vi "FFT.vi"() -> ()   [LabVIEW 2020]
uses:
  <vilib>/rvi/Analysis/measure/FFT/simModelSupport/niFPGA FFT Outside SCTL Sim Properties.ctl
  <vilib>/rvi/Analysis/measure/FFT/simModelSupport/niFPGA FFT Sim Types.ctl
  <vilib>/rvi/Analysis/measure/FFT/simModelSupport/niFpgaFFTSimArithmeticProperties.ctl
  <vilib>/rvi/Analysis/measure/FFT/simModelSupport/niFpgaFFTSimDfxp.ctl
  <vilib>/fxp/LVFixedPointQuantizationPolicyTypeDef.ctl
  <vilib>/rvi/FXPMathLib/FxpAtan2/subVIs/nifxpmath_Atan2_SimConfig.ctl
  <vilib>/rvi/FXPMathLib/FxpSinAndCos/subVIs/nifxpmath_SinAndCos_SimConfig.ctl
  <vilib>/rvi/DataTransferAndStorage/Container/Common/niFpgaContainerGetUniqueNameForEmu.vi
  <vilib>/rvi/DataTransferAndStorage/Container/Common/niFpgaContainerSetEmuInfo.vi
  <vilib>/rvi/eio/common/nirviEmuReportErrorAndStop.vi
  <vilib>/rvi/interface/RandomDataEmulation/niFpgaRandomDataHandleErrors.vi
  <vilib>/rvi/DataTransferAndStorage/Container/Common/niFpgaContainerExecOnDevCompGetState.vi
  <vilib>/rvi/Emulation/niFpgaEmulationIsFPGAContextNoSignature.vi
  <vilib>/rvi/Emulation/niFpgaSctlEmulationGetInTimedLoop.vi
  <vilib>/rvi/errors/niFpgaSetErrorForExecOnDevCompSimple.vi
  <vilib>/rvi/FIFO/Fifo_Resource/nirvififoEmulationSetSize.vi
  <vilib>/rvi/FIFO/Fifo_Resource/nirviFifoEmulationQueueMgr.vi
  <instcachedir>/0/nirviFifoEmulationQueueMgr_E5CAEC123FF24DC58D834DCA3CDAA9B5.lvgen/nirviFifoEmulationQueueMgr_E5CAEC123FF24DC58D834DCA3CDAA9B5_008.vi
  <vilib>/rvi/FIFO/Fifo_Resource/nirvififoEmulationDetermineInputValidOut.vi
  <vilib>/rvi/FIFO/Fifo_Resource/nirvififoEmulationCreateLock.vi
  <vilib>/rvi/Emulation/niFpgaProcessEmulError.vi
  <vilib>/rvi/FIFO/Fifo_Resource/nirvififoEmulationObtainLock.vi
  <vilib>/rvi/FIFO/Fifo_Resource/nirvififoEmulationReleaseLock.vi
  <vilib>/rvi/occurrence/nirviWaitOnOccurrenceBase.vi
  <vilib>/rvi/errors/nirviReportUnexpectedCaseInternalError.vi
  <vilib>/rvi/errors/nirviReportUnexpectedCaseInternalError (U32).vi
  <vilib>/Utility/error.llb/Clear Errors.vi
  <vilib>/rvi/Emulation/niFpgaGetClockAttributes.vi
  <vilib>/rvi/Emulation/niFpgaEmulationReportErrorSimple.vi
  <vilib>/rvi/Analysis/measure/FFT/simModelSupport/niFpgaFFTSimModelOutsideSCTLCore.vi
  <vilib>/rvi/FXPMathLib/FxpAtan2/simVIs/DllFxpAtan2Temp_sub.vi
  <instcachedir>/0/nirviFifoEmulationQueueMgr_E5CAEC123FF24DC58D834DCA3CDAA9B5.lvgen/nirviFifoEmulationQueueMgr_E5CAEC123FF24DC58D834DCA3CDAA9B5_002.vi
  <instcachedir>/0/nirviFifoEmulationQueueMgr_E5CAEC123FF24DC58D834DCA3CDAA9B5.lvgen/nirviFifoEmulationQueueMgr_E5CAEC123FF24DC58D834DCA3CDAA9B5_004.vi
  <vilib>/rvi/Emulation/niFpgaCriticalErrorInLSC.vi
  <vilib>/rvi/FXPMathLib/FxpSinAndCos/simVIs/DllFxpSinAndCosTemp_sub.vi
  <vilib>/rvi/LocalResourceManager/LocalResourceManager.xnode
  <vilib>/rvi/DataTransferAndStorage/Container/XNode/niFpgaContainer.xnode
  <vilib>/rvi/interface/RandomDataEmulation/nirviRandomDataFpgaReadWriteTemplate.vi
  <vilib>/rvi/FIFO/Fifo_Resource/niFpgaFifoEmulationRefIn.vi
  <vilib>/rvi/Analysis/measure/FFT/XNode/niFpgaFFT.xnode
  <vilib>/rvi/FXPMathLib/FxpAtan2/XNode/nifxpmath_Atan2.xnode
  <vilib>/rvi/FXPMathLib/FxpSinAndCos/XNode/nifxpmath_SinAndCos.xnode
panel:
  out "Array":fxp<+/-,33,17>[](array[numeric])
  out "x*y":fxp<+/-,32,16>[](array[numeric])
  out "Numeric 4":i32
  out "Numeric 2":i32
  out "Numeric 3":i32
  out "val":fxp<+,64,48>
  out "n*d":fxp<+,32,16>
  out "size(s)":i32
  out "N":fxp<+/-,18,17>
  in  "n":fxp<+,32,16>
  in  "s (sample rate)":fxp<+,32,16>
  out "Numeric":i32
  # "n=512"
  # "s=51200"
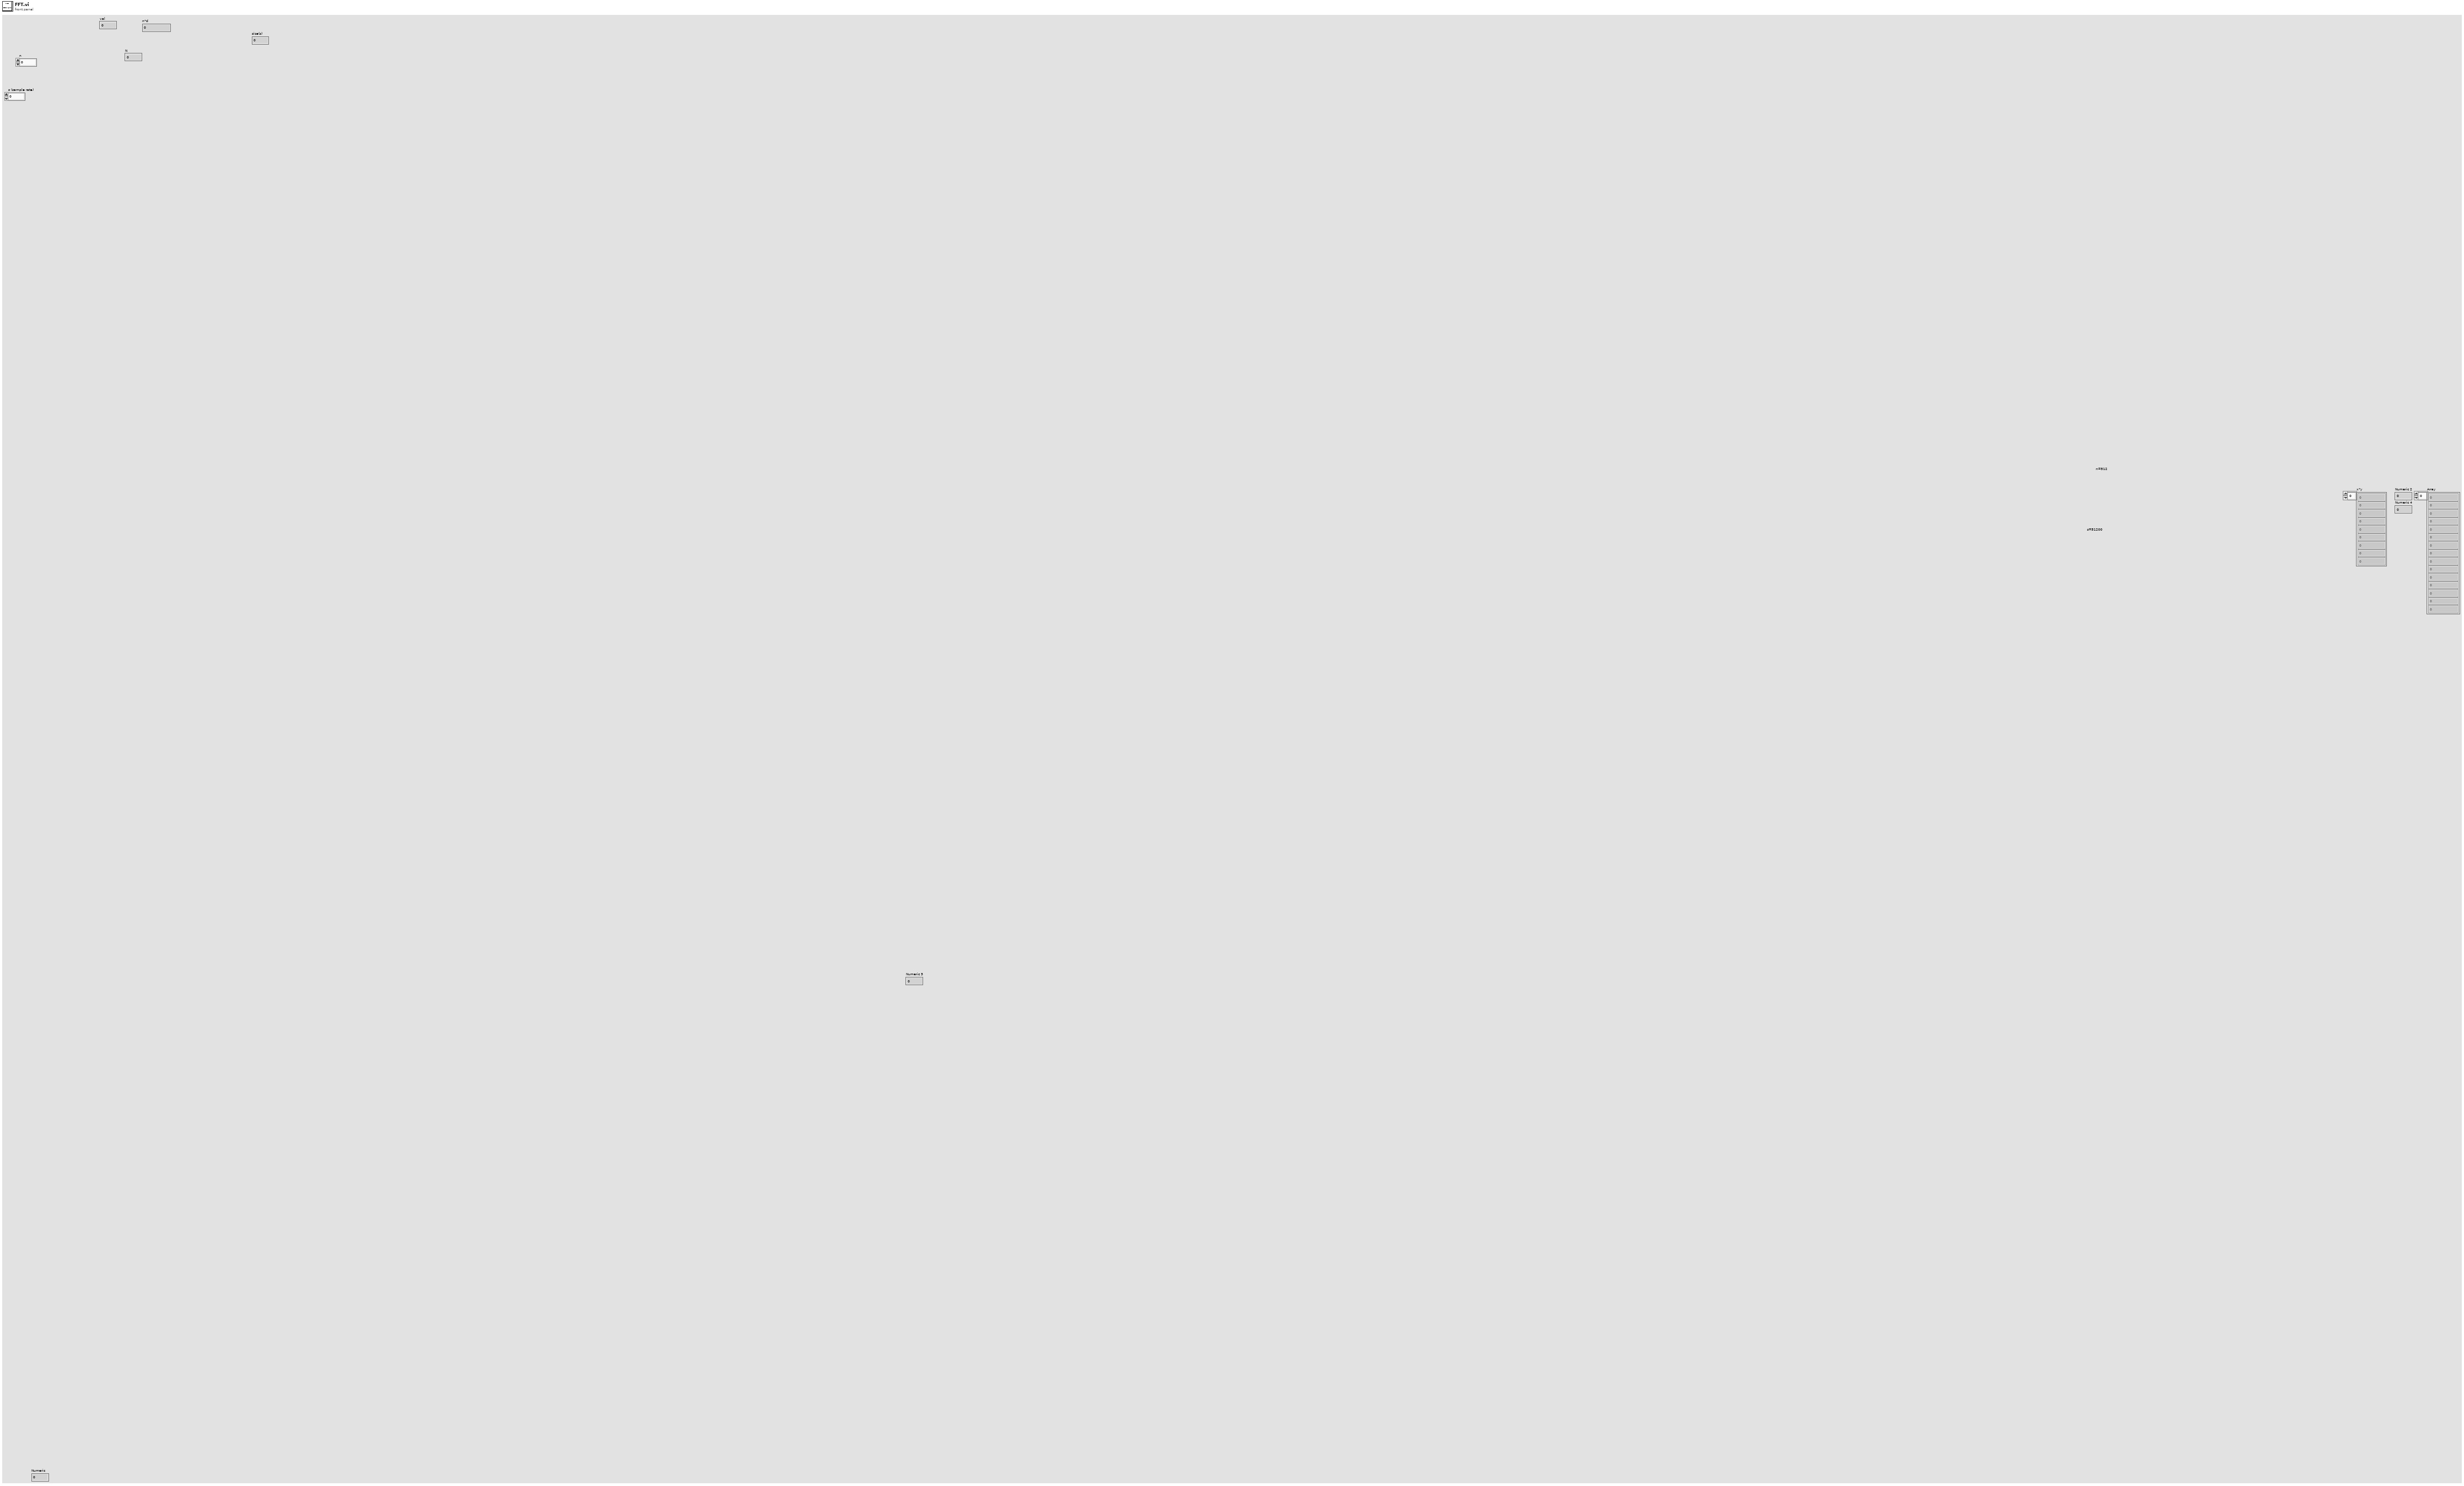
[diagram p1: front panel]
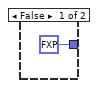
[diagram p2: hidden frame]
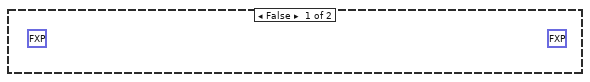
[diagram p3: hidden frame]
diagram:
  (unwired) fxp<+/-,32,16> 0.0
  w3 = 512  # sample rate/input
  w2 = 128  # FFT size
  # "restored_sig += ampli * np.cos(2 * np.pi * (f[j]*Ts * t1 + phase)"
  # "restored_sig += ampli * np.cos(2 * np.pi * (f[j]*Ts * t1 + phase))"
  # ">> frequency interval (delta)>>"
  # "https://www.edn.com/tip-ffts-in-labview-fpga/"
  n1 = xnode "VI-Defined FIFO Configuration"() -> ("FIFO Out"=w12:refnum<k21>)
  n2 = flat-sequence {
    tunnel: w12 -> [w14]
    tunnel: w12 -> [w22]
    tunnel: w11 -> [w21]
    tunnel: w10 -> [w20]
    tunnel: w11 -> [w198]
    tunnel: w10 -> [w197]
    tunnel: w9 -> [w196]
    tunnel: w8 -> [w195]
    tunnel: w9 -> [w229]
    tunnel: w8 -> [w228]
    frame #0 {
      # "data input from host to target"
      n3 = for {
        N: 766 -> [_]
        tunnel: w14 -> [w18]
        i -> [w15]
        n4 = xnode ("FIFO Read")("Timeout"=0) -> ("Element"=w16:fxp<+/-,24,7>)  [unwired: 1 in, 2 out]
        n5 = xnode ("FIFO Write")("Element"=w16, "Timeout"=0, "FIFO In"=w18) -> ()  [unwired: 2 out]
        "Numeric" <- w15
      }
    }
    frame #1 {
      # "FFT based prediction whole process"
      n6 = while {
        tunnel: w22 -> [w32]
        tunnel: w21 -> [w25]
        tunnel: w20 -> [w24]
        tunnel: [w23] -> _
        i -> [w31]
        stop <- w26 stop-if-true
        n7 = flat-sequence {
          tunnel: w32 -> [w36]
          tunnel: [w35] -> w30
          tunnel: [w34] -> w23
          tunnel: w30 -> [w46]
          tunnel: [w45] -> w29
          tunnel: [w44] -> w28
          tunnel: [w43] -> w27
          tunnel: w29 -> [w71]
          tunnel: w28 -> [w70]
          tunnel: w27 -> [w67]
          tunnel: w25 -> [w69]
          tunnel: w24 -> [w68]
          frame #0 {
            w34 = TRUE
            # "signal input through FIFO iteam"
            n8 = case shown="True" w34 {
              tunnel: w36 -> [_ w40]
              tunnel: [fxp<+/-,24,7> 0.0 ("Element") w38] -> w35
              frame False {
              }
              frame True {
                n9 = xnode ("FIFO Write")("Timeout"=0, "FIFO In"=w40) -> ("Element"=w38:fxp<+/-,24,7>)  [unwired: 2 out]
              }
            }
          }
          frame #1 {
            # "FFT function for getting real and imaginary values"
            n10 = xnode ("FIFO Write")("Element"=w46, "Timeout"=0) -> ()  [unwired: 1 in, 2 out]
            n11 = xnode ("FFT")("real data in"=w46, "reset"=FALSE) -> ("real data out"=w45:fxp<+/-,32,15>, "imaginary data out"=w44:fxp<+/-,32,15>, "output valid"=w43:bool)  [unwired: 1 in, 1 out]
          }
          frame #2 {
            # "measuring magnitude, phase and frequencies"
            n12 = case shown="True" w67 {
              tunnel: w70 -> [_ w74]
              tunnel: w71 -> [_ w73]
              tunnel: w69 -> [_ w78]
              tunnel: w68 -> [_ w75]
              frame False {
                (unwired) fxp<+/-,32,16> 0.0
                (unwired) fxp<+/-,32,16> 0.0
              }
              frame True {
                # "magnitude=root (x^2+y^2)\nwhere, x=real and y=imag"
                # "phase=arctan(img(Y)/real(x))\nhere in FPGA we don't have arctan\nso m odified arctan=cos/sine\nphase=cos(z)/sine(z), where z=(y/x)"
                n13 = Square(x=w73) -> (x^2=w82:fxp<+,63,29>)
                n14 = Square(x=w74) -> (x^2=w77:fxp<+,63,29>)
                n15 = xnode "High Throughput Inverse Tangent (2 Input)"("y"=w74, "x"=w73) -> ("atan2(y,x) (pi)"=w72:fxp<+/-,16,2>)
                n16 = xnode ("FIFO Write")("Element"=w72, "Timeout"=0) -> ()  [unwired: 1 in, 2 out]
                n17 = xnode ("FIFO Write")("Element"=w72, "Timeout"=0, "FIFO In"=w75) -> ()  [unwired: 2 out]
                n18 = Add(x=w82, y=w77) -> (x+y=w81:fxp<+,64,30>)
                n19 = Square Root(x=w81) -> (sqrt(x)=w80:fxp<+/-,32,16>)
                n20 = xnode ("FIFO Write")("Element"=w80, "Timeout"=0) -> ()  [unwired: 1 in, 2 out]
                n21 = xnode ("FIFO Write")("Element"=w80, "Timeout"=0, "FIFO In"=w78) -> ()  [unwired: 2 out]
              }
            }
          }
        }
        n22 = Greater?(x=w31, y=766 ("Timeout")) -> (0:w26:bool)
      }
    }
    frame #2 {
    }
    frame #3 {
      n23 = flat-sequence {
        tunnel: ["n"] -> w132
        tunnel: ["s (sample rate)"] -> _
        tunnel: ["n"] -> _
        tunnel: ["s (sample rate)"] -> w131
        tunnel: ["n"] -> w130
        tunnel: ["n"] -> w129
        tunnel: [w139] -> w128
        tunnel: w132 -> [w138]
        tunnel: w131 -> [w137]
        tunnel: [w137] -> w127
        tunnel: w130 -> [w136]
        tunnel: [w136] -> w126
        tunnel: w129 -> [w135]
        tunnel: [w135] -> w125
        tunnel: w128 -> [w151]
        tunnel: [w149] -> w124
        tunnel: w127 -> [w148]
        tunnel: [w148] -> w123
        tunnel: w126 -> [w147]
        tunnel: [w147] -> w122
        tunnel: w125 -> [w146]
        tunnel: [w146] -> w121
        tunnel: [w162] -> w120
        tunnel: [w158] -> _
        tunnel: w124 -> [w158]
        tunnel: w123 -> [w161]
        tunnel: [w161] -> w119
        tunnel: w122 -> [w160]
        tunnel: w121 -> [w159]
        tunnel: [w159] -> w118
        tunnel: [w158] -> w117
        tunnel: w120 -> [w178]
        tunnel: w119 -> [w177]
        tunnel: [w177] -> w116
        tunnel: [w176] -> w115
        tunnel: [w176] -> w114
        tunnel: w118 -> [w175]
        tunnel: [w175] -> w113
        tunnel: w117 -> [w174]
        tunnel: w116 -> [w184]
        tunnel: w115 -> [w183]
        tunnel: w114 -> [w182]
        tunnel: w113 -> [w181]
        frame #0 {
          # "n=windowlength\ns= sample rate\nd=inverserse of sampling rate in numpy\ns=1/d"
        }
        frame #1 {
          # "N=(n-1)//2+1"
          n24 = Subtract(x=w138, y=fxp<+,1,1> 1.0) -> (x-y=w143:fxp<+/-,33,17>)
          n25 = Divide(x=w143, y=fxp<+,1,2> 2.0) -> (x/y=w144:fxp<+/-,34,16>)
          n26 = Round Toward -Infinity(1:w144) -> (0:w145:fxp<+/-,16,16>)
          n27 = Add(x=w145, y=fxp<+,1,1> 1.0) -> (x+y=w139:fxp<+/-,18,17>)
          "N" <- w139
        }
        frame #2 {
          # "p1=arange(0,N,dtype=int)"
          n28 = To Long Integer(number=w151) -> (32bit integer=w152:i32)
          n29 = for {
            N: w152 -> [_]
            shift-right: [w153] -> _
            shift-left: fxp<+,1,1> 0.0 -> [w155]
            shift-right: [w156] -> w149
            shift-left: _ -> [w157]
            n30 = Increment(x=w155) -> (x+1=w154:fxp<+/-,33,33>)
            n31 = Build Array (concatenate)(w157, w155) -> (w156:fxp<+/-,32,32>[])
            n32 = To Long Integer(number=w154) -> (32bit integer=w153:i32)
          }
        }
        frame #3 {
          # "p2 =arange(-(n//2),0,dtype=int)"
          n33 = Divide(x=w160, y=fxp<+,1,2> 2.0) -> (x/y=w165:fxp<+,33,15>)
          n34 = Round Toward -Infinity(1:w165) -> (0:w167:fxp<+,15,15>)
          n35 = To Long Integer(number=w167) -> (32bit integer=w166:i32)
          n36 = for {
            N: w166 -> [_]
            shift-right: [w169] -> _
            shift-left: fxp<+,1,1> 0.0 -> [w171]
            shift-right: [w172] -> w168
            shift-left: _ -> [w173]
            n37 = Decrement(x=w171) -> (x-1=w170:fxp<+/-,33,33>)
            n38 = Build Array (concatenate)(w173, w171) -> (w172:fxp<+/-,32,32>[])
            n39 = To Long Integer(number=w170) -> (32bit integer=w169:i32)
          }
          n40 = Reverse 1D Array(array=w168) -> (reversed array=w162:fxp<+/-,32,32>[])
        }
        frame #4 {
          # "results=empty(n,int)\nresults[:N]=p1\nresults[N:]=p2"
          n41 = Insert Into Array(array=w174, new element=w178) -> (w176:fxp<+/-,32,32>[])  [unwired: 1 in]
        }
        frame #5 {
          # "val=1/(n*d)\nf=results*val"
          n42 = Divide(x=w181, y=w184) -> (x/y=w187:fxp<+,64,32>)
          "n*d" <- w187
          n43 = Array Size(array=w183) -> (size(s)=w186:i32)
          n44 = Divide(x=fxp<+,32,32> 1.0, y=w187) -> (x/y=w188:fxp<+,32,16>)
          "val" <- w188
          n45 = Round Toward -Infinity(1:w188) -> (0:w189:fxp<+,16,16>)
          n46 = for {
            N: w186 -> [_]
            tunnel: w189 -> [w193]
            tunnel: [w191] -> w180 mode=indexing
            tunnel: w182 -> [w192] mode=indexing
            n47 = Multiply(x=w192, y=w193) -> (x*y=w191:fxp<+/-,32,16>)
            n48 = xnode ("FIFO Write")("Element"=w191, "Timeout"=0) -> ()  [unwired: 1 in, 2 out]
          }
          n49 = Array Size(array=w180) -> (size(s)=→"size(s)":i32)
        }
      }
    }
    frame #4 {
      w194 = fxp<+/-,32,16>[] [128.0, 132.0, 136.0, 252.0, 256.0, 260.0, 380.0, 384.0, 388.0, -128.0, -132.0, -136.0, -252.0, -256.0, -260.0, -380.0, -384.0, -388.0]  # selective frequencies
      w203 = 512  # sample rate/input
      w204 = 128  # FFT size
      # "GOAL:\n1. build a list of frequencies\n2. use the list for building a forloop"
      # "What done?\n1. make a array of 18 frequencies\n2. devide frequency array with frequency interval(delta) to get its sample points\n3. to get specific magnitude and phase of the specific frequency use index array through a for loop\n5. get magnitude and phase of that 28 frequencies."
      # ">> frequency interval (delta)>>"
      # "collect specific frequencies"
      n50 = for {
        N: 512 -> [_]
        tunnel: [w224] -> w202 mode=indexing
        tunnel: [w223] -> w201 mode=indexing
        tunnel: w198 -> [w222]
        tunnel: w197 -> [w221]
        n51 = xnode ("FIFO Write")("Timeout"=0, "FIFO In"=w222) -> ("Element"=w223:fxp<+/-,32,16>)  [unwired: 2 out]
        n52 = xnode ("FIFO Write")("Timeout"=0, "FIFO In"=w221) -> ("Element"=w224:fxp<+/-,16,2>)  [unwired: 2 out]
      }
      n53 = To Fixed-Point(number=w203) -> (fixed-point=w206:fxp<+/-,32,32>)  [unwired: 1 in]
      n54 = To Fixed-Point(number=w204) -> (fixed-point=w205:fxp<+/-,32,32>)  [unwired: 1 in]
      n55 = Divide(x=w206, y=w205) -> (x/y=w207:fxp<+/-,32,16>)
      n56 = Divide(x=w194, y=w207) -> (x/y=w208:fxp<+/-,32,16>[])
      n57 = To Long Integer(number=w208) -> (32bit integer=w200:i32[])
      n58 = for {
        tunnel: w200 -> [w219] mode=indexing
        tunnel: w202 -> [w218]
        tunnel: w201 -> [w217]
        tunnel: w196 -> [w214]
        tunnel: w195 -> [w209]
        i -> [w220]
        n59 = Index Array(array=w217, index=w219) -> (element=w211:fxp<+/-,32,16>)
        n60 = Index Array(array=w218, index=w219) -> (element=w213:fxp<+/-,16,2>)
        n61 = xnode ("FIFO Write")("Element"=w211, "Timeout"=0, "FIFO In"=w209) -> ()  [unwired: 2 out]
        n62 = xnode ("FIFO Write")("Element"=w211, "Timeout"=0) -> ()  [unwired: 1 in, 2 out]
        n63 = xnode ("FIFO Write")("Element"=w213, "Timeout"=0) -> ()  [unwired: 1 in, 2 out]
        n64 = xnode ("FIFO Write")("Element"=w213, "Timeout"=0, "FIFO In"=w214) -> ()  [unwired: 2 out]
        "Numeric 3" <- w220
      }
    }
    frame #5 {
      # "1. build extended time(t1)\n2. use restored signal equation to get each signal of each frequency\n3. use a transpose 2D array > forloop to sum all frequencies and get restored signal."
      # "extended time"
      n65 = for {
        N: 18 -> [_]
        tunnel: w229 -> [w249]
        tunnel: w228 -> [w251]
        w230 = fxp<+/-,32,16>[] [128.0, 132.0]  # selective frequencies
        w231 = fxp<+/-,32,16>[] [1.0, 2.0, 3.0, 4.0, 5.0, 6.0]  # Ts building
        # "2pi"
        n66 = xnode ("FIFO Write")("Timeout"=0, "FIFO In"=w251) -> ()  [unwired: 3 out]
        n67 = Reverse 1D Array(array=w230) -> (reversed array=w232:fxp<+/-,32,16>[])
        n68 = for {
          N: 18 -> [_]
          tunnel: w249 -> [w292]
          tunnel: [w291] -> w234 mode=indexing
          i -> [w290]
          n69 = xnode ("FIFO Write")("Timeout"=0, "FIFO In"=w292) -> ("Element"=w291:fxp<+/-,32,16>)  [unwired: 2 out]
          "Numeric 4" <- w290
        }
        n70 = Multiply(x=2, y=3) -> (x*y=w245:i32)
        n71 = To Fixed-Point(number=w245) -> (fixed-point=w244:fxp<+/-,32,32>)  [unwired: 1 in]
        n72 = Multiply(x=w232, y=w244) -> (x*y=w246:fxp<+/-,64,48>[])
        n73 = Divide(x=fxp<+,1,1> 1.0, y=fxp<+,5,16> 51200.0) -> (x/y=w247:fxp<+,1,-15>)
        n74 = Multiply(x=w246, y=w247) -> (x*y=w237:fxp<+/-,64,32>[])
        n75 = Multiply(x=w231, y=w237) -> (x*y=w236:fxp<+/-,32,16>[])
        "x*y" <- w236
        n76 = for {
          N: 6 -> [_]
          tunnel: w236 -> [w252] mode=indexing
          tunnel: w234 -> [w254] mode=indexing
          tunnel: [w253] -> w233 mode=indexing
          n77 = Add(x=w252, y=w254) -> (x+y=w253:fxp<+/-,33,17>)
        }
        "Array" <- w233
        n78 = for {
          N: 18 -> [_]
          tunnel: w233 -> [w259] mode=indexing
          tunnel: [w258] -> w238 mode=indexing
          i -> [w257]
          n79 = xnode "High Throughput Sine & Cosine"("x (pi)"=w259) -> ("cos(x)"=w258:fxp<+/-,32,2>)  [unwired: 1 out]
          "Numeric 2" <- w257
        }
        n80 = for {
          tunnel: w238 -> [w255] mode=indexing
          n81 = xnode ("FIFO Write")("Element"=w255, "Timeout"=0) -> ()  [unwired: 1 in, 2 out]
        }
      }
    }
  }
  n82 = xnode "VI-Defined FIFO Configuration"() -> ("FIFO Out"=w11:refnum<k21>)
  n83 = xnode "VI-Defined FIFO Configuration"() -> ("FIFO Out"=w10:refnum<k21>)
  n84 = xnode "VI-Defined FIFO Configuration"() -> ("FIFO Out"=w8:refnum<k21>)
  n85 = xnode "VI-Defined FIFO Configuration"() -> ("FIFO Out"=w9:refnum<k21>)
  n86 = To Fixed-Point(number=w3) -> (fixed-point=w6:fxp<+/-,32,32>)  [unwired: 1 in]
  n87 = To Fixed-Point(number=w2) -> (fixed-point=w7:fxp<+/-,32,32>)  [unwired: 1 in]
  n88 = Divide(x=w6, y=w7) -> (x/y=w4:fxp<+/-,32,16>)
  n89 = feedback #1() -> (w5:fxp<+/-,32,16>)  [unwired: 1 in]
  n90 = Add(x=w5, y=w4) -> (x+y=w1:fxp<+/-,32,16>)
  n91 = feedback-in #1(w1) -> ()
